vi "Curl_Height_Body.vi"(0 "Wm":dbl format="%#_13g", 5 "Hm":dbl format="%#_13g", 7 "Curl Gap":dbl format="%#_13g", 9 "cos_net":dbl format="%#_13g", 11 "sin_net":dbl format="%#_13g") -> (4 "H":dbl)   [LabVIEW 2019, in "Algorithm.lvclass"]
uses:
  FrameworkOverrides/Algorithm.lvclass
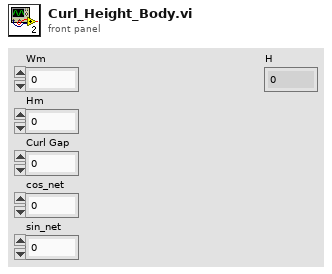
[diagram p1: front panel]
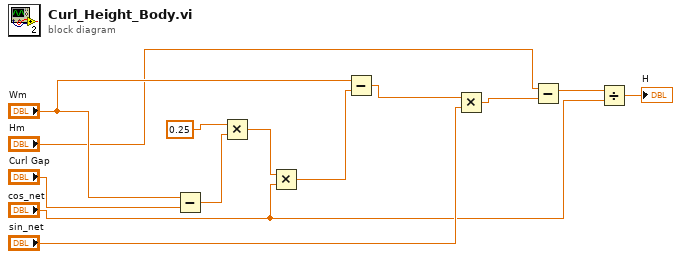
[diagram p0: block diagram]
diagram:
  n1 = Subtract(x="Wm", y="Curl Gap") -> (x-y=w11:dbl)
  n2 = Multiply(x=0.25, y=w11) -> (x*y=w10:dbl)
  n3 = Multiply(x=w10, y="cos_net") -> (x*y=w9:dbl)
  n4 = Subtract(x="Wm", y=w9) -> (x-y=w7:dbl)
  n5 = Multiply(x=w7, y="sin_net") -> (x*y=w4:dbl)
  n6 = Subtract(x="Hm", y=w4) -> (x-y=w3:dbl)
  n7 = Divide(x=w3, y="cos_net") -> (x/y=→"H":dbl)
